vi "test Acyclic Loopback Value Overflow.vi"(8 "error in":errorcluster, 11 "TestCase in":refnum<class "Octal Loopback.lvclass">) -> (0 "error out":errorcluster, 3 "TestCase out":refnum<class "Octal Loopback.lvclass">)   [LabVIEW 2020, in "Octal Loopback.lvclass"]
uses:
  Octal Loopback.lvclass
  C:/Program Files (x86)/National Instruments/LabVIEW 2020/vi.lib/NI/VeriStand Custom Device Testing Tools/VeriStandTestCase/VeriStandTestCase.lvclass
  <vilib>/numeric/Random Number (Range) U64.vi
  <vilib>/numeric/sub_Random U32.vi
  <vilib>/NI VeriStand/Execution/Workspace/NI VeriStand - Set Multiple Channel Values.vi
  <vilib>/addons/_JKI Toolkits/VI Tester/TestCase.llb/TestCase.lvclass
  <vilib>/NI VeriStand/Execution/Workspace/NI_VS Workspace ExecutionAPI.lvlib
  <vilib>/NI/VeriStand Custom Device Testing Tools/VeriStandTestUtilities/VeriStandTestUtilities.lvlib
  C:/Program Files (x86)/National Instruments/LabVIEW 2020/vi.lib/addons/_JKI Toolkits/VI Tester/TestCase.llb/TestCase.lvclass
  C:/Users/nitest/Desktop/Git 2020/niveristand-ballard-arinc429-custom-device/Source/Custom Device Support/Tests/System/Octal Loopback/Octal Loopback.lvclass
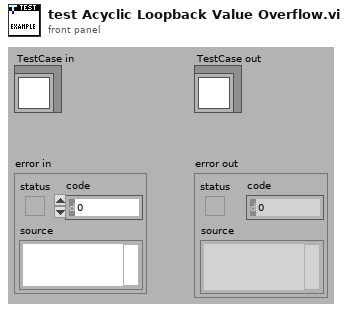
[diagram p1: front panel]
types:
  T1 = typedef "NI_VS Workspace ExecutionAPI.lvlib/WorkspaceAPI.ctl" = refnum<k24>
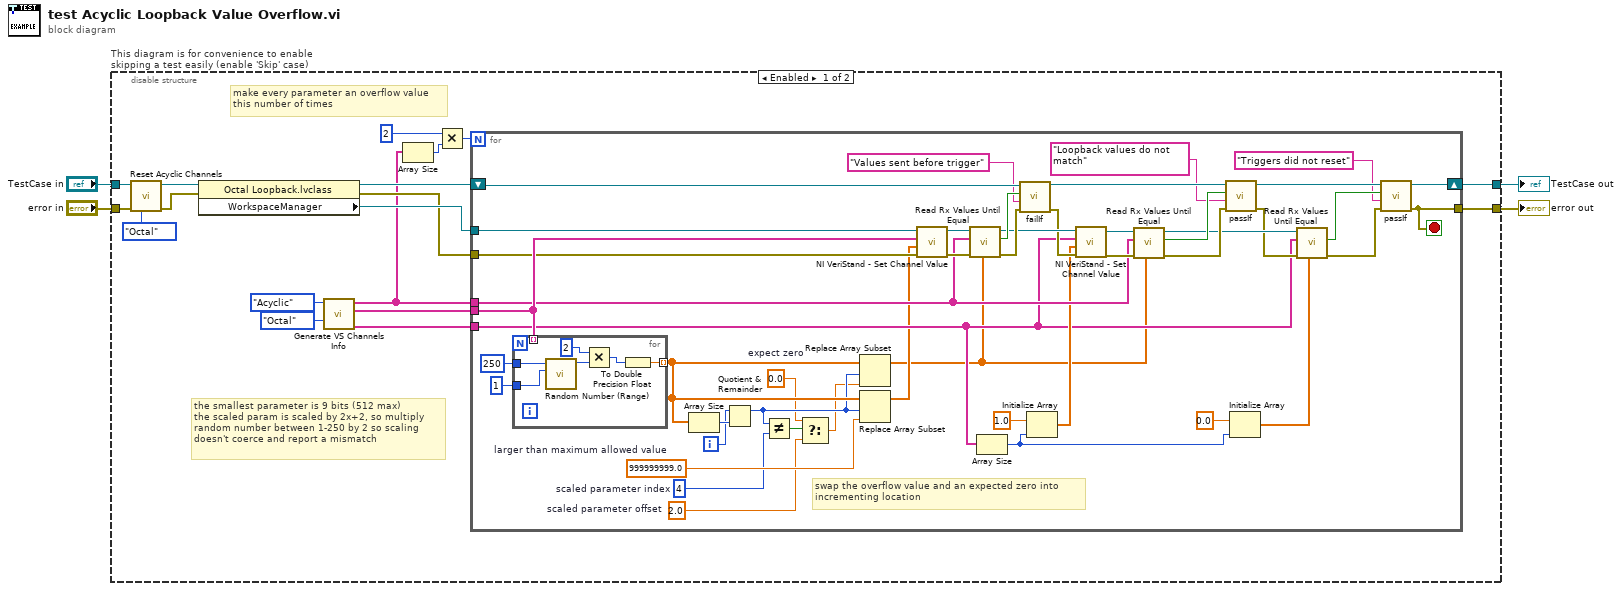
[diagram p0: block diagram]
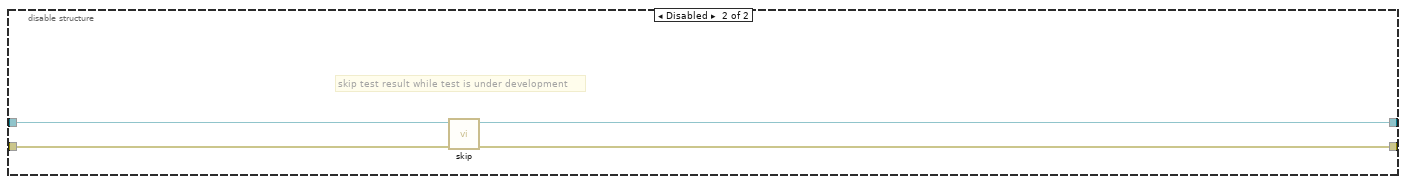
[diagram p2: hidden frame]
diagram:
  n1 = disable-structure "This diagram is for convenience to enable skipping a test easily (enable 'Skip' case)" shown="Enabled" {
    disable-tunnel: "TestCase in" -> [w7 w78]
    disable-tunnel: [w18 w76] -> w1
    disable-tunnel: [w17 w77] -> w3
    disable-tunnel: "error in" -> [w19 w75]
    frame Enabled {
      # "make every parameter an overflow value\nthis number of times"
      # "the smallest parameter is 9 bits (512 max)\nthe scaled param is scaled by 2x+2, so multiply \nrandom number between 1-250 by 2 so scaling\ndoesn't coerce and report a mismatch"
      n2 = call "Reset Acyclic Channels.vi"("error in (no error)"=w19, "Label Format (Decimal)"=enum16{"Decimal", "Octal"}."Octal", "reference in"=w7) -> ("error out"=w9:errorcluster, "reference out"=w8:refnum<class "Octal Loopback.lvclass">)  [unwired: 7 in]
      n3 = property class="Octal Loopback.lvclass"(reference=w8, error in=w9) -> (reference out=w20:refnum<class "Octal Loopback.lvclass">, error out=w21:errorcluster, "WorkspaceManager"=w22:T1)
      n4 = call "Generate VS Channels Info.vi"("Label Format (Decimal)"=enum16{"Decimal", "Octal"}."Octal", "Transfer Type"=enum16{"Acyclic", "Scheduled"}."Acyclic") -> ("Tx Trigger Channels Array"=w15:string[], "Tx Channels Array"=w16:string[], "Rx Channels Array"=w11:string[])  [unwired: 5 in, 2 out]
      n5 = Array Size(array=w11) -> (size(s)=w12:i32)
      n6 = Multiply(x=2, y=w12) -> (x*y=w14:i32)
      n7 = for {
        N: w14 -> [_]
        tunnel: w11 -> [w54]
        tunnel: w22 -> [w66]
        tunnel: w21 -> [w59]
        tunnel: w16 -> [w65]
        shift-right: [w48] -> w18
        shift-left: w20 -> [w61]
        tunnel: [w50] -> w17
        tunnel: w15 -> [w39]
        i -> [w31]
        stop <- w50 stop-if-true
        w28 = 2.0  # scaled parameter offset
        w25 = 4  # scaled parameter index
        w27 = 0.0  # expect zero
        w34 = 999999999.0  # larger than maximum allowed value
        # "swap the overflow value and an expected zero into \nincrementing location"
        n8 = for {
          tunnel: [w73] -> w32 mode=indexing
          tunnel: u64 250 ("upper bound (100)") -> [w72]
          tunnel: u64 1 ("upper bound (100)") -> [w71]
          tunnel: w65 -> [_] mode=indexing
          n9 = call-poly <vilib>:"Random Number (Range).vi"("lower bound (0)"=w71, "upper bound (100)"=w72) -> ("number"=w74:u64)  [unwired: 9 in]
          n10 = Multiply(x=u64 2, y=w74) -> (x*y=w70:u64)
          n11 = To Double Precision Float(number=w70) -> (double precision float=w73:dbl)
        }
        n12 = Array Size(array=w32) -> (size(s)=w33:i32)
        n13 = Quotient & Remainder(x=w31, y=w33) -> (x-y*floor(x/y)=w29:i32)  [unwired: 1 out]
        n14 = Not Equal?(x=w29, y=w25) -> (x != y?=w30:bool)
        n15 = Select(t=w27, s=w30, f=w28) -> (s? t:f=w26:dbl)
        n16 = Replace Array Subset(array=w32, new element=w26, index=w29) -> (w23:dbl[])
        n17 = Replace Array Subset(array=w32, new element=w34, index=w29) -> (w35:dbl[])
        n18 = call-poly <vilib>:"NI VeriStand - Set Channel Value.vi"("error in (no error)"=w59, "Values"=w35, "Channels"=w65, "WorkspaceManager in"=w66) -> ("error out"=w62:errorcluster, "WorkspaceManager out"=w64:T1)  [unwired: 6 in]
        n19 = call <vilib>:"Read Rx Values Until Equal.vi"("expected values"=w23, "error in"=w62, "Rx aliases"=w54, "workspace manager in"=w64) -> ("error out"=w63:errorcluster, "values equal expected"=w60:bool, "workspace manager out"=w58:T1)  [unwired: 5 in]
        n20 = Array Size(array=w39) -> (size(s)=w36:i32)
        n21 = call-dynamic "failIf.vi"("error in (no error)"=w63, "message (\"\")"="Values sent before trigger" ("message (\"\")"), "fail"=w60, "TestCase in"=w61) -> ("error out"=w57:errorcluster, "TestCase out"=w51:refnum<class "Octal Loopback.lvclass">)  [unwired: 6 in]
        n22 = Initialize Array(1.0, w36) -> (w40:dbl[])
        n23 = call-poly <vilib>:"NI VeriStand - Set Channel Value.vi"("error in (no error)"=w57, "Values"=w40, "Channels"=w39, "WorkspaceManager in"=w58) -> ("error out"=w55:errorcluster, "WorkspaceManager out"=w56:T1)  [unwired: 6 in]
        n24 = call <vilib>:"Read Rx Values Until Equal.vi"("expected values"=w23, "error in"=w55, "Rx aliases"=w54, "workspace manager in"=w56) -> ("error out"=w52:errorcluster, "values equal expected"=w53:bool, "workspace manager out"=w46:T1)  [unwired: 5 in]
        n25 = call-dynamic "passIf.vi"("error in (no error)"=w52, "message (\"\")"="Loopback values do not match" ("message (\"\")"), "pass"=w53, "TestCase in"=w51) -> ("error out"=w45:errorcluster, "TestCase out"=w49:refnum<class "Octal Loopback.lvclass">)  [unwired: 6 in]
        n26 = Initialize Array(0.0, w36) -> (w37:dbl[])
        n27 = call <vilib>:"Read Rx Values Until Equal.vi"("expected values"=w37, "error in"=w45, "Rx aliases"=w39, "workspace manager in"=w46) -> ("error out"=w44:errorcluster, "values equal expected"=w47:bool)  [unwired: 5 in, 1 out]
        n28 = call-dynamic "passIf.vi"("error in (no error)"=w44, "message (\"\")"="Triggers did not reset" ("message (\"\")"), "pass"=w47, "TestCase in"=w49) -> ("error out"=w50:errorcluster, "TestCase out"=w48:refnum<class "Octal Loopback.lvclass">)  [unwired: 6 in]
      }
    }
    frame Disabled {
      # "skip test result while test is under development"
      n29 = call <vilib>:"skip.vi"("error in (no error)"=w75, "TestCase in"=w78) -> ("error out"=w77:errorcluster, "TestCase out"=w76:refnum<class "Octal Loopback.lvclass">)  [unwired: 8 in]
    }
  }
  "error out" <- w3
  "TestCase out" <- w1
